vi "TestExec.Init Config Files at Launch.vi"(8 "error in":errorcluster, 10 "Station Name":string, 11 "Working Dir":path) -> (0 "error out":errorcluster)   [LabVIEW 2018]
uses:
  <vilib>/KATE/Files/File Utils.lvlib
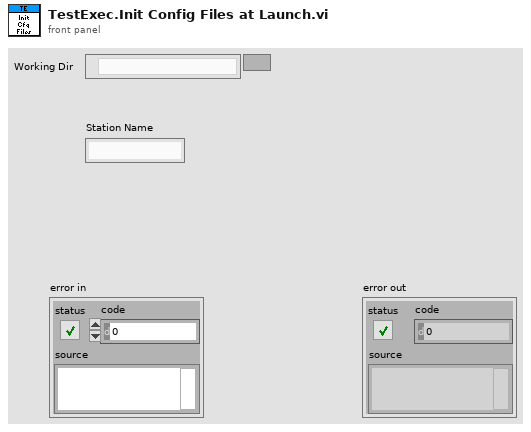
[diagram p1: front panel]
types:
  T1 = enum32{"invalid app kind", "Development System", "Run Time System", "Student Edition", "Embedded LabVIEW", "Evaluation", "Custom"}
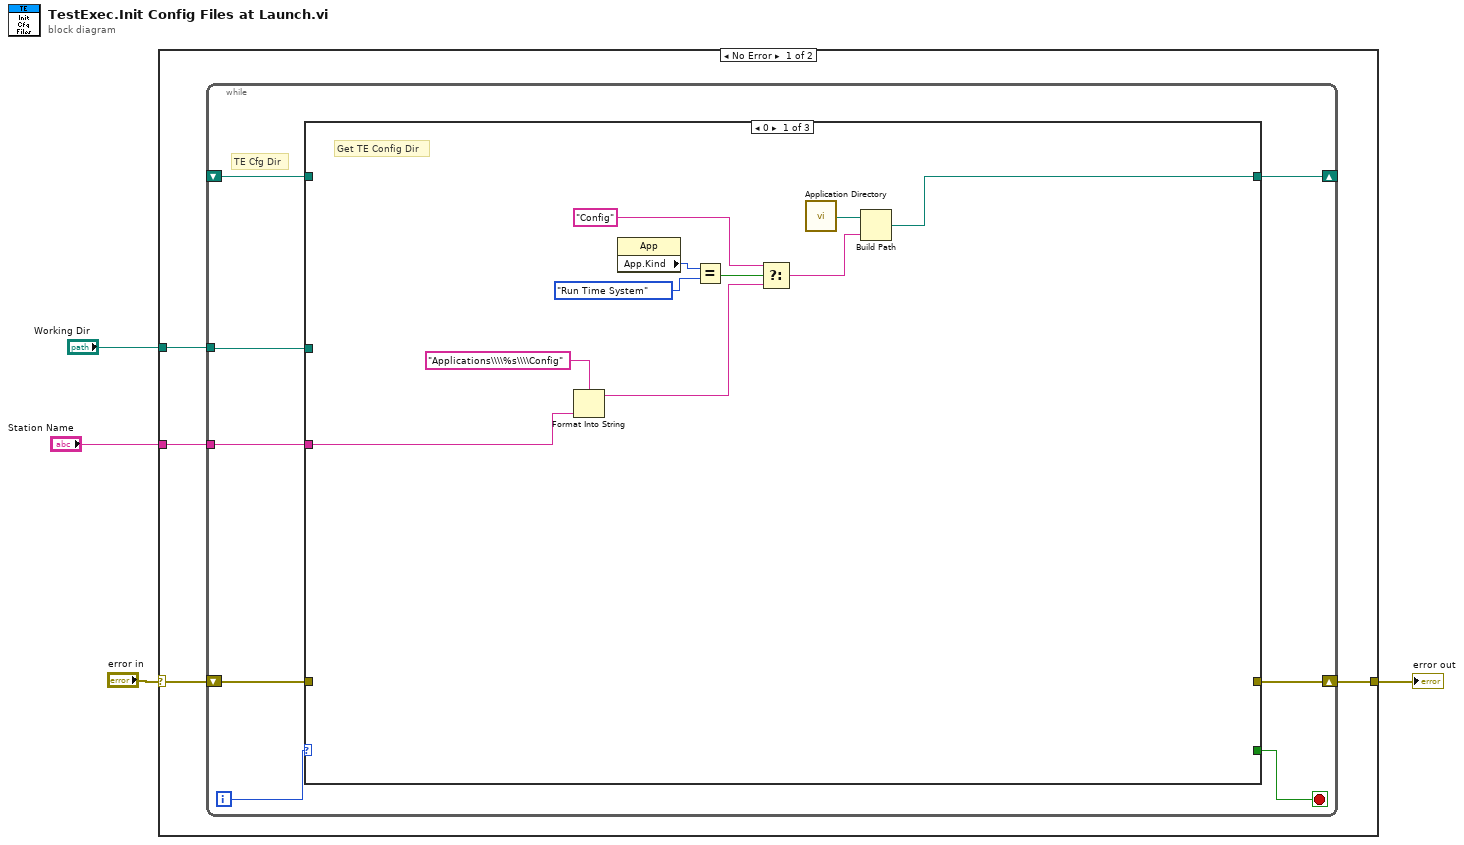
[diagram p0: block diagram]
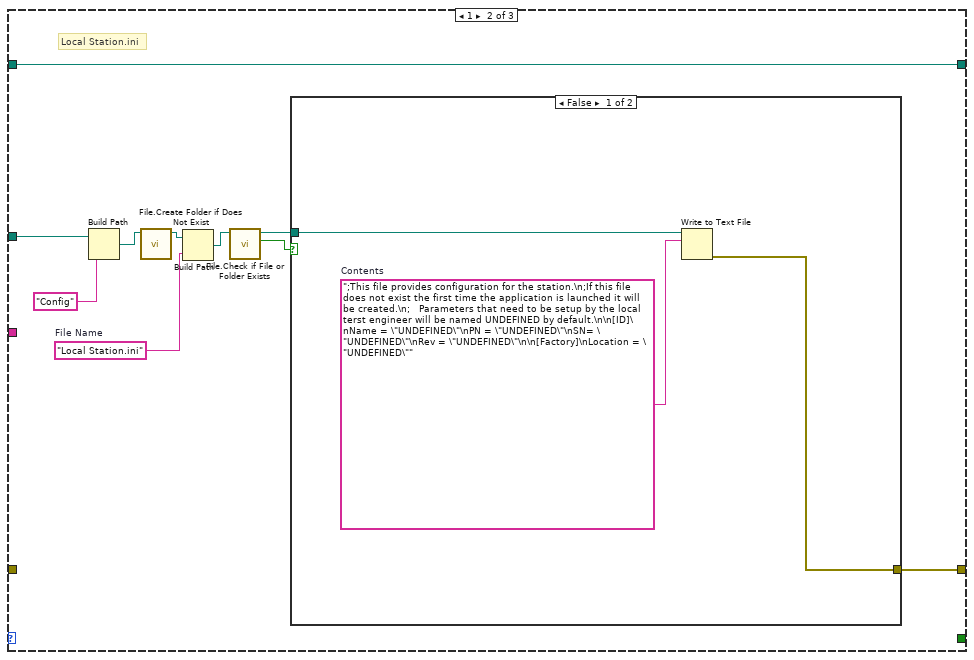
[diagram p2: hidden frame]
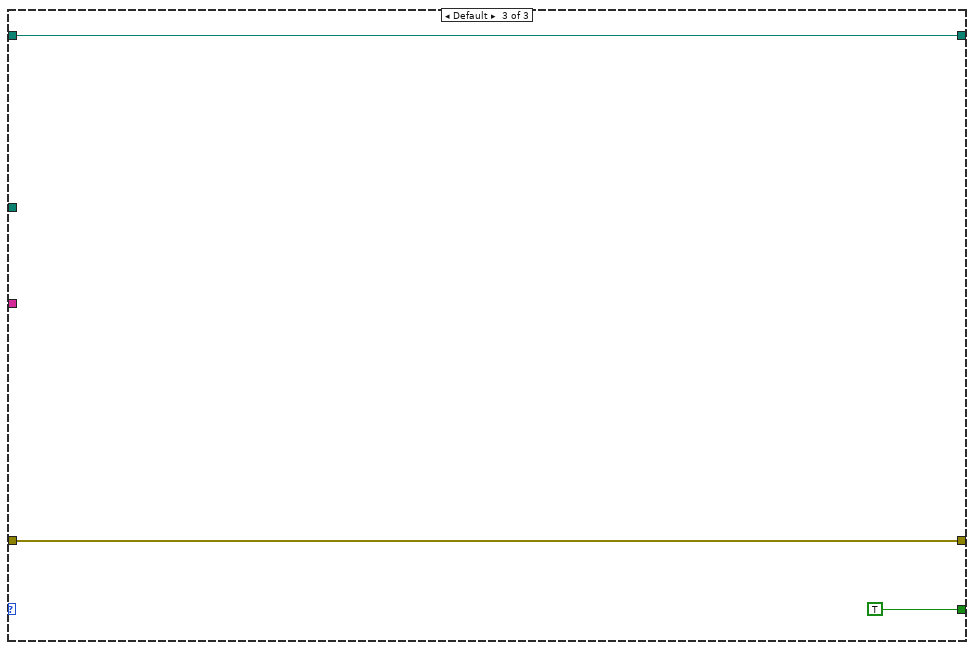
[diagram p4: hidden frame]
diagram:
  n1 = case shown="No Error" "error in" {
    selector: "error in" -> [w8 w43]
    tunnel: [w7 w43] -> w3
    tunnel: "Working Dir" -> [w6 _]
    tunnel: "Station Name" -> [w5 _]
    frame No Error {
      n2 = while {
        shift-right: [w13] -> w7
        shift-left: w8 -> [w14]
        tunnel: w6 -> [w12]
        tunnel: w5 -> [w11]
        shift-right: [w9] -> _
        shift-left: _ -> [w10]
        i -> [w16]
        stop <- w15 stop-if-true
        # "TE Cfg Dir"
        n3 = case shown="0" w16 {
          tunnel: [_ _ TRUE] -> w15
          tunnel: w14 -> [_ _ w41]
          tunnel: [_ w28 w41] -> w13
          tunnel: w12 -> [_ w35 _]
          tunnel: w11 -> [w17 _ _]
          tunnel: w10 -> [_ w27 w40]
          tunnel: [w20 w27 w40] -> w9
          frame 0 {
            # "Get TE Config Dir"
            n4 = Format Into String(format string="Applications\\\\%s\\\\Config", w17) -> (resulting string=w18:string)  [unwired: 2 in, 1 out]
            n5 = property class="App"() -> ("App.Kind"=w23:T1)  [unwired: 2 in, 2 out]
            n6 = Equal?(x=w23, y=T1."Run Time System" ("Application:Kind")) -> (x = y?=w25:bool)
            n7 = Select(t="Config", s=w25, f=w18) -> (s? t:f=w24:string)
            n8 = call <vilib>:"Application Directory.vi"() -> ("Application Directory"=w26:path)
            n9 = Build Path(base path=w26, name or relative path=w24) -> (appended path=w20:path)
          }
          frame 1 {
            w34 = "Local Station.ini"  # File Name
            # "Local Station.ini"
            n10 = Build Path(base path=w35, name or relative path="Config" ("section")) -> (appended path=w31:path)
            n11 = call <vilib>:"File.Create Folder if Does Not Exist.vi"("Path"=w31) -> ("Dup Path"=w30:path)  [unwired: 8 in, 2 out]
            n12 = Build Path(base path=w30, name or relative path=w34) -> (appended path=w33:path)
            n13 = call <vilib>:"File.Check if File or Folder Exists.vi"("Path"=w33) -> ("Exists"=w29:bool, "Dup Path"=w32:path)  [unwired: 6 in, 3 out]
            n14 = case shown="False" w29 {
              tunnel: w32 -> [w38 _]
              tunnel: [w37 _] -> w28
              frame False {
                w39 = ";This file provides configuration for the station.\n;If this file does not exist the first time the application is launched it will be created.\n;   Parameters that need to be setup by the local terst engineer will be named UNDEFINED by default.\n\n[ID]\nName = \"UNDEFINED\"\nPN = \"UNDEFINED\"\nSN= \"UNDEFINED\"\nRev = \"UNDEFINED\"\n\n[Factory]\nLocation = \"UNDEFINED\""  # Contents
                n15 = Write to Text File(file (use dialog)=w38, text=w39) -> (error out=w37:errorcluster)  [unwired: 2 in, 2 out]
              }
              frame True {
                # "Do Nothing"
              }
            }
          }
          frame Default {
          }
        }
      }
    }
    frame Error {
    }
  }
  "error out" <- w3
